vi "Serial Comm.vi"(6 "error in":errorcluster, 8 "Data Out":string, 9 "VISA resource name in":refnum<visa-resource-name>) -> (0 "error out":errorcluster, 1 "Number of Bytes at Serial Port":u32, 2 "Data In":string, 3 "VISA resource name out":refnum<visa-resource-name>)   [LabVIEW 2017]
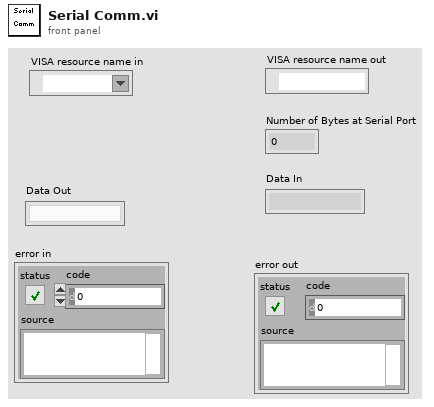
[diagram p1: front panel]
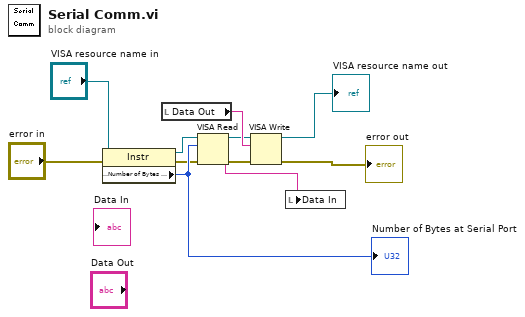
[diagram p0: block diagram]
diagram:
  n1 = property class="Instr"(reference="VISA resource name in", error in="error in") -> (reference out=w3:refnum<visa-resource-name>, error out=w4:errorcluster, "Serial Settings:Number of Bytes at Serial Port"=w5:u32)
  "Number of Bytes at Serial Port" <- w5
  n2 = local read "Data Out"() -> (w9:string)
  n3 = VISA Read(VISA resource name=w3, byte count=w5, error in (no error)=w4) -> (VISA resource name out=w6:refnum<visa-resource-name>, read buffer=w8:string, error out=w7:errorcluster)  [unwired: 1 out]
  n4 = VISA Write(VISA resource name=w6, write buffer=w9, error in (no error)=w7) -> (VISA resource name out=→"VISA resource name out":refnum<visa-resource-name>, error out=→"error out":errorcluster)  [unwired: 1 out]
  n5 = local write "Data In"(w8) -> ()
